vi "OpenVI.vi"(0 "vi path":path) -> ()   [LabVIEW 2014]
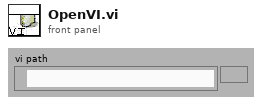
[diagram p1: front panel]
types:
  T1 = enum32{"Invalid", "Standard", "Closed", "Hidden", "Minimized", "Maximized"}
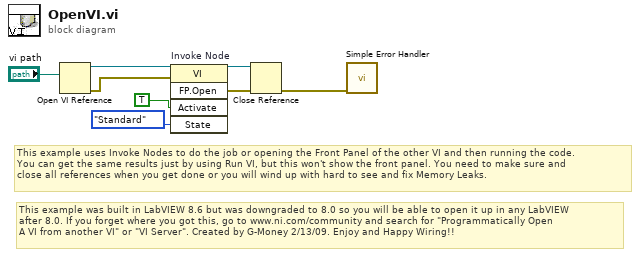
[diagram p0: block diagram]
diagram:
  # "This example was built in LabVIEW 8.6 but was downgraded to 8.0 so you will be able to open it up in any LabVIEW \nafter 8.0. If you forget where you got this, go to www.ni.com/community and search for \"Programmatically Open \nA VI from another VI\" or \"VI Server\". Created by G-Money 2/13/09. Enjoy and Happy Wiring!!"
  # "This example uses Invoke Nodes to do the job or opening the Front Panel of the other VI and then running the code. \nYou can get the same results just by using Run VI, but this won't show the front panel. You need to make sure and \nclose all references when you get done or you will wind up with hard to see and fix Memory Leaks."
  n1 = Open VI Reference(vi path="vi path") -> (vi reference=w7:refnum<vi>, error out=w6:errorcluster)  [unwired: 1 in, 4 out]
  n2 = invoke on="Invoke Node" class="VI" method="FP.Open"(reference=w7, error in=w6, "Activate"=TRUE ("Activate?"), "State"=T1."Standard") -> (reference out=w2:refnum<vi>, error out=w1:errorcluster)  [unwired: 1 in, 3 out]
  n3 = Close Reference(reference=w2, error in (no error)=w1) -> (error out=w5:errorcluster)
  n4 = call <vilib>:"Simple Error Handler.vi"("error in (no error)"=w5) -> ()  [unwired: 1 in, 8 out]
